vi "Measure Multi.vi"(7 "Config for Immediate Measure?(T)":bool=TRUE, 8 "error in (no error)":errorcluster, 9 "Max Time (-1ms)":i32=-1, 10 "Measurements to Acquire(1)":i32=1 min=0, 11 "DMM Driver in":refnum<class "DMM Driver.lvclass">) -> (0 "error out":errorcluster, 2 "Measurements":dbl[](array[numeric]), 3 "DMM Driver out":refnum<class "DMM Driver.lvclass">)   [LabVIEW 2020, in "DMM.lvlib" / "DMM Driver.lvclass"]
doc: "Perform multiple measurement on the DMM. \nTimeout should not result in errors.\nMeasurements should only contain actual completed measurements."
uses:
  DMM Driver.lvclass
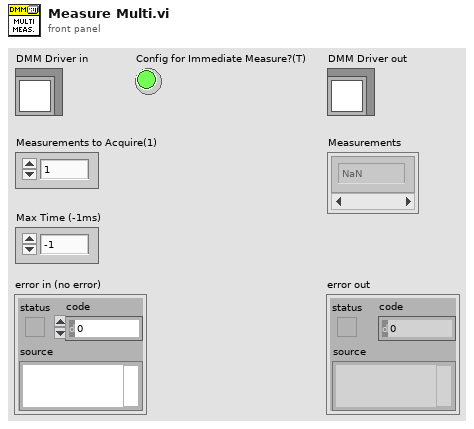
[diagram p1: front panel]
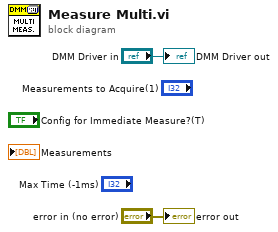
[diagram p0: block diagram]
diagram:
  "error out" <- "error in (no error)"
  "DMM Driver out" <- "DMM Driver in"
